vi "Get_Data.vi"(0 "Add in":refnum<class "Add.lvclass">, 11 "Error In":errorcluster) -> (4 "Add out":refnum<class "Add.lvclass">, 15 "Error Out":errorcluster)   [LabVIEW 2020, in "Add.lvclass"]
uses:
  Add.lvclass
  Arithmetic_Operations/Arithmetic_Operations.lvclass
  Add.lvclass/Add.ctl
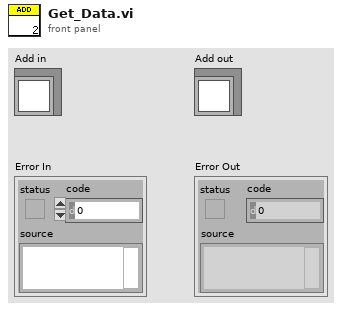
[diagram p1: front panel]
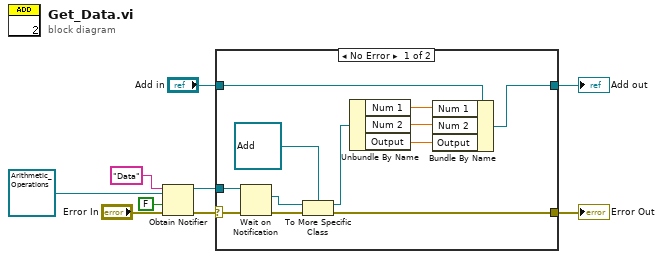
[diagram p0: block diagram]
diagram:
  n1 = Obtain Notifier(name (unnamed)="Data", notification data type=refnum<class "Arithmetic_Operations.lvclass"> refnum ("Arithmetic_Operations.lvclass"), create if not found? (T)=FALSE, error in (no error)="Error In") -> (notifier out=w5:refnum<notifier>, error out=w3:errorcluster)  [unwired: 1 out]
  n2 = case shown="No Error" w3 {
    selector: w3 -> [w16 w23]
    tunnel: [w13 w23] -> w9
    tunnel: [w20 w22] -> w7
    tunnel: "Add in" -> [w21 w22]
    tunnel: w5 -> [w14 _]
    frame No Error {
      n3 = Wait on Notification(notifier=w14, error in (no error)=w16) -> (notification=w12:refnum<class "Arithmetic_Operations.lvclass">, error out=w15:errorcluster)  [unwired: 2 in, 2 out]
      n4 = To More Specific Class(target class=refnum<class "Add.lvclass"> refnum ("Add.lvclass"), reference=w12, error in=w15) -> (specific class reference=w11:refnum<class "Add.lvclass">, error out=w13:errorcluster)
      n5 = Unbundle By Name(w11) -> ("Num 1"=w19:dbl, "Num 2"=w18:dbl, "Output"=w17:dbl)
      n6 = Bundle By Name(cluster=w21, "Num 1"=w19, "Num 2"=w18, "Output"=w17) -> (w20:refnum<class "Add.lvclass">)
    }
    frame Error {
    }
  }
  "Error Out" <- w9
  "Add out" <- w7
